vi "LookupIndicies.vi"(9 "Lookup String":string, 11 "Report Header Indicies":string[][](array[string])) -> (1 "Column":i32, 2 "Row":i32)   [LabVIEW 2015, in "csv-formatter.lvclass"]
uses:
  csv-formatter.lvclass
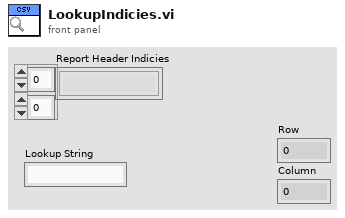
[diagram p1: front panel]
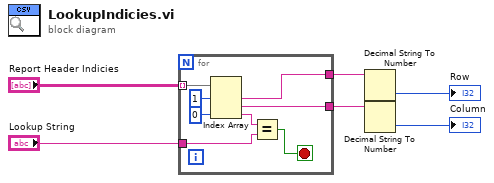
[diagram p0: block diagram]
diagram:
  n1 = for {
    tunnel: "Lookup String" -> [w10]
    tunnel: "Report Header Indicies" -> [w14] mode=indexing
    tunnel: [w8] -> w3
    tunnel: [w7] -> w4
    stop <- w9 stop-if-true
    n2 = Index Array(array=w14, index #1=1 ("index"), index #3=0 ("index")) -> (element #1=w8:string, element #2=w7:string, element #3=w11:string)  [unwired: 1 in]
    n3 = Equal?(x=w11, y=w10) -> (x = y?=w9:bool)
  }
  n4 = Decimal String To Number(string=w3) -> (number=→"Row":i32)  [unwired: 2 in, 1 out]
  n5 = Decimal String To Number(string=w4) -> (number=→"Column":i32)  [unwired: 2 in, 1 out]
